vi "Max Tipper Angle.vi"() -> ()   [LabVIEW 2012]
panel:
  in  "Extra Sting Angle":dbl
  in  "Max Stinger Angle":dbl
  in  "Max Tipper Angle":dbl=1.56
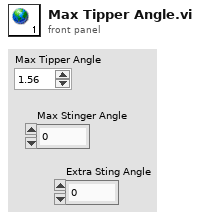
[diagram p1: front panel]
diagram:
